vi "UDP Data Link - RTMs - Import from XML.vi"(8 "error in (no error)":errorcluster, 11 "Node Ptr":u64 format="%.0x") -> (0 "error out":errorcluster)   [LabVIEW 2015, in "UDP Data Link System Explorer.lvlib"]
uses:
  UDP Data Link System Explorer.lvlib
  TypeDefs/UDP Data Link - TypeDefs - Section Info.ctl
  Shared/UDP Data Link Global.vi
  Shared/UDP Data Link Shared.lvlib
  <vilib>/NI Veristand/Custom Device Tools/Custom Device Utility Library/Custom Device Utility Library.lvlib
panel:
  in  "Tag":string
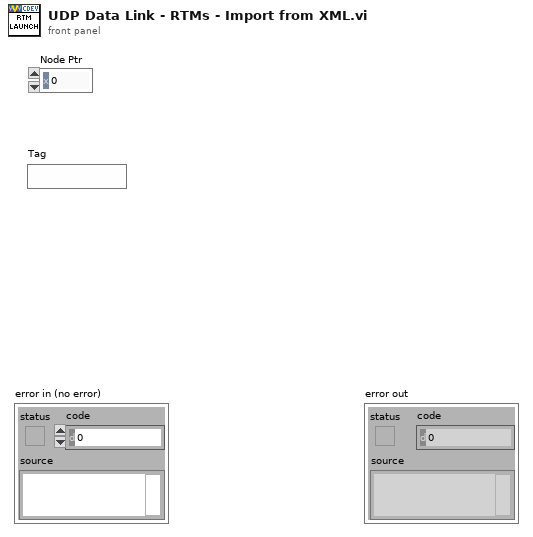
[diagram p1: front panel]
types:
  T1 = typedef "UDP Data Link System Explorer.lvlib/UDP Data Link - TypeDefs - Section Info.ctl" = cluster{"Section GUID":string, "Channel Refs":string, "Channel Names":string, "Channel Paths":string}
  T2 = typedef "UDP Data Link System Explorer.lvlib/UDP Data Link - TypeDefs - XML Channel.ctl" = cluster{"Channel Name":string, "Data Type":u16, "Description":string, "Unit":string}
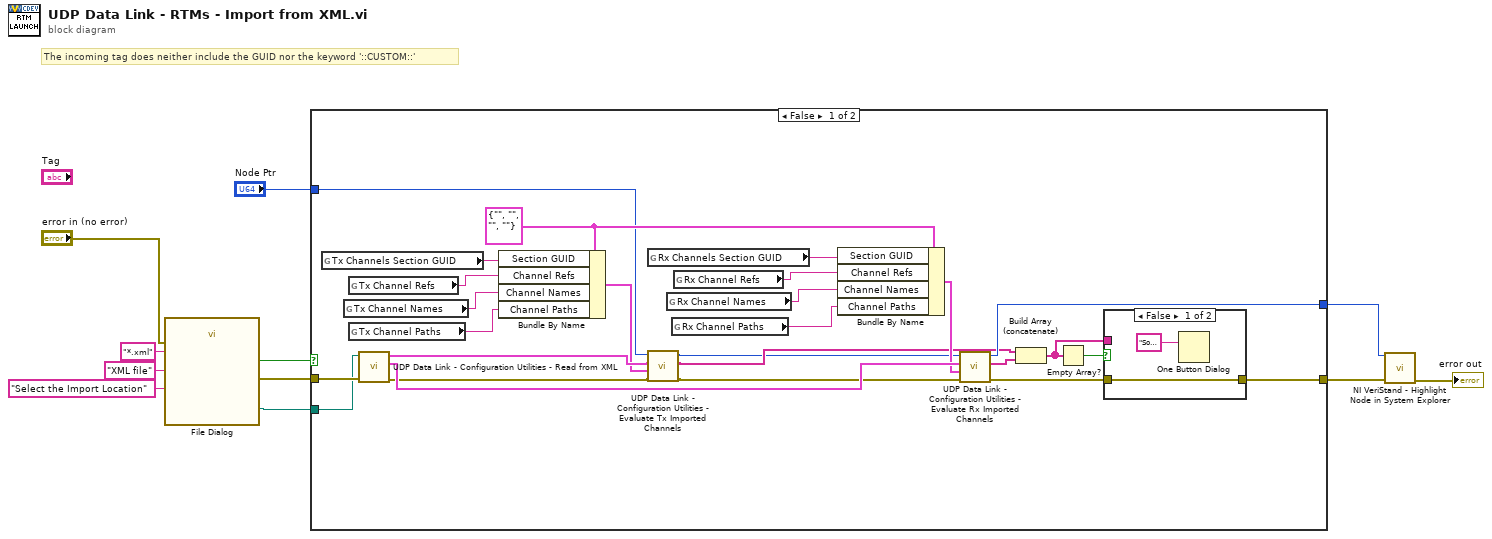
[diagram p0: block diagram]
diagram:
  # "The incoming tag does neither include the GUID nor the keyword '::CUSTOM::'"
  n1 = call "File Dialog"("prompt"="Select the Import Location", "error in"="error in (no error)", "pattern (all files)"="*.xml", "pattern label"="XML file") -> ("selected path"=w5:path, "cancelled"=w7:bool, "error out"=w6:errorcluster)  [unwired: 8 in, 1 out]
  n2 = case shown="False" w7 {
    tunnel: w6 -> [w37 w42]
    tunnel: w5 -> [w36 _]
    tunnel: [w32 w42] -> w4
    tunnel: "Node Ptr" -> [w18 w41]
    tunnel: [w19 w41] -> w1
    frame False {
      w26 = T1 {"Section GUID"="", "Channel Refs"="", "Channel Names"="", "Channel Paths"=""} ("Section Info")
      n3 = global read "UDP Data Link Global.vi" "Tx Channels Section GUID"() -> (w30:string)
      n4 = global read "UDP Data Link Global.vi" "Tx Channel Names"() -> (w28:string)
      n5 = global read "UDP Data Link Global.vi" "Tx Channel Refs"() -> (w29:string)
      n6 = global read "UDP Data Link Global.vi" "Tx Channel Paths"() -> (w27:string)
      n7 = call "UDP Data Link - Configuration Utilities - Read from XML.vi"("error in (no error)"=w37, "path to XML document"=w36) -> ("error out"=w15:errorcluster, "Rx Channel Info"=w35:T2[], "Tx Channel Info"=w17:T2[])  [unwired: 7 in]
      n8 = Bundle By Name(cluster=w26, "Section GUID"=w30, "Channel Refs"=w29, "Channel Names"=w28, "Channel Paths"=w27) -> (w16:T1)
      n9 = global read "UDP Data Link Global.vi" "Rx Channels Section GUID"() -> (w25:string)
      n10 = call "UDP Data Link - Configuration Utilities - Evaluate Tx Imported Channels.vi"("error in (no error)"=w15, "Section Info"=w16, "Channel Info Array"=w17, "Node Ptr in"=w18) -> ("error out"=w14:errorcluster, "Invalid Channels"=w13:string[], "Node Ptr out"=w12:u64)  [unwired: 5 in]
      n11 = global read "UDP Data Link Global.vi" "Rx Channel Names"() -> (w23:string)
      n12 = global read "UDP Data Link Global.vi" "Rx Channel Paths"() -> (w22:string)
      n13 = global read "UDP Data Link Global.vi" "Rx Channel Refs"() -> (w24:string)
      n14 = Bundle By Name(cluster=w26, "Section GUID"=w25, "Channel Refs"=w24, "Channel Names"=w23, "Channel Paths"=w22) -> (w21:T1)
      n15 = call "UDP Data Link - Configuration Utilities - Evaluate Rx Imported Channels.vi"("error in (no error)"=w14, "Section Info"=w21, "Channel Info Array"=w35, "Node Ptr in"=w12) -> ("error out"=w33:errorcluster, "Invalid Channels"=w34:string[], "Node Ptr out"=w19:u64)  [unwired: 5 in]
      n16 = Build Array (concatenate)(w13, w34) -> (w20:string[])
      n17 = Empty Array?(array=w20) -> (empty?=w31:bool)
      n18 = case shown="False" w31 {
        tunnel: w33 -> [w39 w40]
        tunnel: [w39 w40] -> w32
        tunnel: w20 -> [_ _]
        frame False {
          n19 = One Button Dialog(message="Some channels were unable to be added because they do not exist in the current system definition.") -> ()  [unwired: 1 in, 1 out]
        }
        frame True {
        }
      }
    }
    frame True {
    }
  }
  n20 = call <vilib>:"NI VeriStand - Highlight Node in System Explorer.vi"("error in (no error)"=w4, "Item Ref in"=w1) -> ("error out"=→"error out":errorcluster)  [unwired: 8 in, 1 out]
